vi "LVClass_Camera get image sequence.vi"(0 "Camera in":refnum<class "Camera.lvclass">, 5 "Image array":refnum<class "Image.lvclass">[](array[class]), 11 "error in (no error)":errorcluster) -> (4 "Camera out":refnum<class "Camera.lvclass">, 6 "Image array (dup)":refnum<class "Image.lvclass">[](array[class]), 15 "error out":errorcluster)   [LabVIEW 2020, in "Camera.lvclass"]
doc: "Ask camera for array_size captures and retrieve images array (Synchronous mode\n- Blocking).\n\n--------------------------------------------------------------------------------\n\n<B>CameraIn</B> : Camera object.\n\n<B>CameraOut</B> : Camera object.\n\n<B>image_array_size</B> : Captured sequence length (number of cImage).\n\n<B>image_array</B> : Captured sequence as cImage array.\n\n<B>ErrorIn</B> : Error\n\n<B>ErrorOut</B> : Error"
uses:
  Camera.lvclass
  Image.lvclass
  Camera.lvclass/Camera.ctl
  LVClass_Image read Image Compat ptr.vi
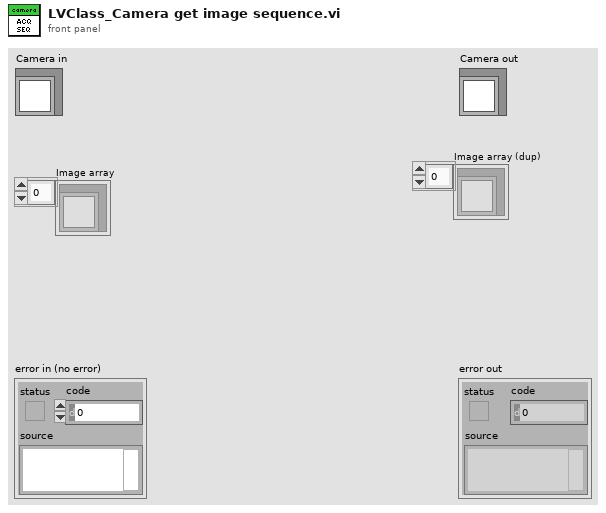
[diagram p1: front panel]
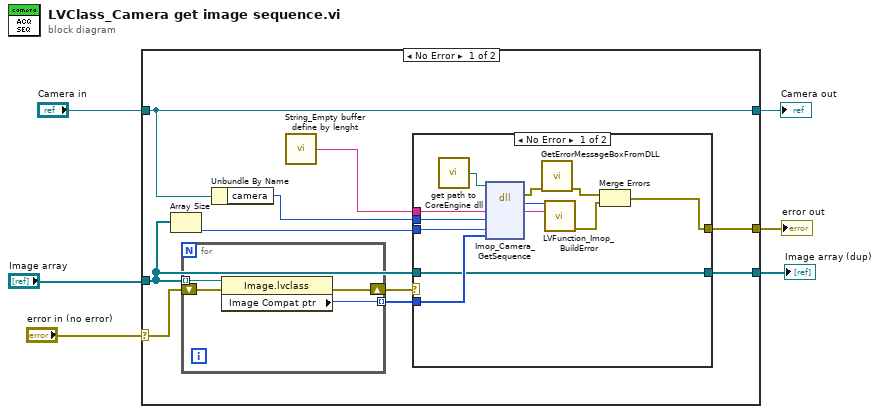
[diagram p0: block diagram]
diagram:
  n1 = case shown="No Error" "error in (no error)" {
    selector: "error in (no error)" -> [w13 w37]
    tunnel: [w15 w37] -> w5
    tunnel: [w9 w36] -> w3
    tunnel: "Camera in" -> [w9 w36]
    tunnel: "Image array" -> [w7 w35]
    tunnel: [w10 w35] -> w1
    frame No Error {
      n2 = Array Size(array=w7) -> (size(s)=w11:i32)
      n3 = for {
        tunnel: w7 -> [w33] mode=indexing
        tunnel: [w34] -> w14 mode=indexing
        shift-right: [w31] -> w12
        shift-left: w13 -> [w32]
        n4 = property class="Image.lvclass"(reference=w33, error in=w32) -> (error out=w31:errorcluster, "Image Compat ptr"=w34:i32)  [unwired: 1 out]
      }
      n5 = Unbundle By Name(w9) -> ("camera"=w8:i32)
      n6 = call "String_Empty buffer define by lenght.vi"() -> ("Empty buffer"=w16:string)  [unwired: 1 in]
      n7 = case shown="No Error" w12 {
        selector: w12 -> [_ w30]
        tunnel: w16 -> [w28 _]
        tunnel: [w17 w30] -> w15
        tunnel: w8 -> [w25 _]
        tunnel: w14 -> [w24 _]
        tunnel: w11 -> [w21 _]
        tunnel: w7 -> [w20 w29]
        tunnel: [w20 w29] -> w10
        frame No Error {
          n8 = call "get path to CoreEngine dll.vi"() -> ("path to c_interface_vc100.dll"=w23:path)  [unwired: 12 in, 3 out]
          n9 = dll-call lib="D:/soft/HASO_v3/SVN_trunk/ImOpCoreEngine4_LV2011/DLLs/c_interface_vc100.dll" fn="Imop_Camera_GetSequence"(path in=w23, "message"=w28, "camera"=w25, "array_size"=w21, "HASO_image_array"=w24) -> (error out=w22:errorcluster, "return type"=w26:i32, "message"=w27:string)  [unwired: 5 in, 1 out]
          n10 = call "GetErrorMessageBoxFromDLL.vi"("error IN"=w22) -> ("error OUT"=w19:errorcluster)  [unwired: 10 in]
          n11 = call "LVFunction_Imop_BuildError.vi"("code"=w26, "String to Prepend to source (\"\")"=w27) -> ("error out"=w18:errorcluster)  [unwired: 13 in]
          n12 = Merge Errors(w19, w18) -> (w17:errorcluster)
        }
        frame Error {
        }
      }
    }
    frame Error {
    }
  }
  "error out" <- w5
  "Camera out" <- w3
  "Image array (dup)" <- w1
